vi "Convert Step Index to Section Name.vi"(11 "Step Index":i32) -> (3 "Section Name":string)   [LabVIEW 2020, in "MacroAssert.lvlib"]
doc: "Converts <B>Step Index</B> to an associated section name."
uses:
  MacroAssert.lvlib
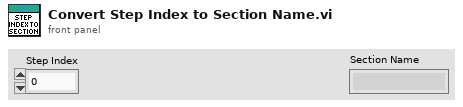
[diagram p1: front panel]
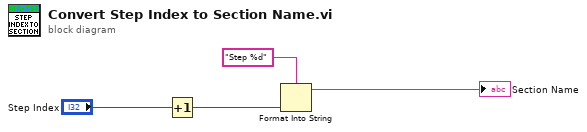
[diagram p0: block diagram]
diagram:
  n1 = Increment(x="Step Index") -> (x+1=w1:i32)
  n2 = Format Into String(format string="Step %d", w1) -> (resulting string=→"Section Name":string)  [unwired: 2 in, 1 out]
